vi "Process pos.vi"(6 "Fs":dbl, 9 "LSB":dbl, 10 "New gyro read":u16, 11 "Pos ref":refnum<vi>) -> ()   [LabVIEW 2017]
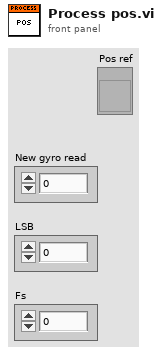
[diagram p1: front panel]
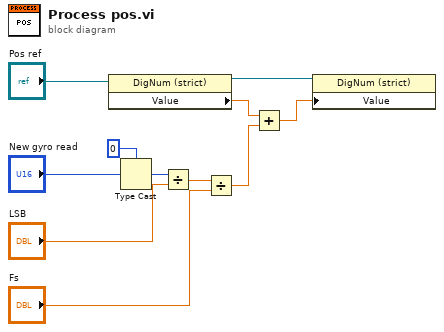
[diagram p0: block diagram]
diagram:
  n1 = property on="Property Node" class="DigNum (strict)"(reference="Pos ref") -> (reference out=w1:refnum<vi>, "Value"=w3:dbl)  [unwired: 1 in, 1 out]
  n2 = Type Cast(type=i16 0, x="New gyro read") -> (*(type *) &x=w7:i16)
  n3 = Divide(x=w7, y="LSB") -> (x/y=w9:dbl)
  n4 = Divide(x=w9, y="Fs") -> (x/y=w11:dbl)
  n5 = Add(x=w3, y=w11) -> (x+y=w2:dbl)
  n6 = property on="Property Node" class="DigNum (strict)"(reference=w1, "Value"=w2) -> ()  [unwired: 1 in, 2 out]
